vi "MGI Bezier Optimizer.vi"(0 "Sample Points":dbl[][](array[numeric]) format="%.2f", 1 "Substitution Matrix":dbl[][](array[numeric]) format="%.2f", 2 "Constant Vector":dbl[](array[numeric]) format="%.2f", 3 "Accuracy Limit":dbl=1e-08 format="%.3e", 4 "Start Vector":dbl[](array[numeric]) format="%.2f") -> (5 "Bezier Points":dbl[][](array[numeric]) format="%.2f", 6 "Log":dbl[][](array[numeric]) format="%.2f")   [LabVIEW 2020]
doc: "Modification of Downhill Simplex nD to perform modelling calculation and provide an interactive display.\n\nAuthored by David A. Moore\nsupport@mooregoodideas.com\nwww.mooregoodideas.com\n\nCopyright (c) 2010, Moore Good Ideas, Inc.\n\nAll rights reserved.\n\nRedistribution and use in source and binary forms, with or without modification, are permitted provided that the following conditions are met:\n\n * Redistributions of source code must retain the above copyright notice, this list of conditions and the following disclaimer.\n * Redistributions in binary form must reproduce the above copyright notice, this list of conditions and the following disclaimer in the documentation and/or other materials provided with the distribution.\n * Neither the name of Moore Good Ideas, Inc. nor the names of its contributors may be used to endorse or promote products derived from this software without specific prior written permission.\n\nTHIS SOFTWARE IS PROVIDED BY THE COPYRIGHT HOLDERS AND CONTRIBUTORS \"AS IS\" AND ANY EXPRESS OR IMPLIED WARRANTIES, INCLUDING, BUT NOT LIMITED TO, THE IMPLIED WARRANTIES OF MERCHANTABILITY AND FITNESS FOR A PARTICULAR PURPOSE ARE DISCLAIMED. IN NO EVENT SHALL THE COPYRIGHT OWNER OR CONTRIBUTORS BE LIABLE FOR ANY DIRECT, INDIRECT, INCIDENTAL, SPECIAL, EXEMPLARY, OR CONSEQUENTIAL DAMAGES (INCLUDING, BUT NOT LIMITED TO, PROCUREMENT OF SUBSTITUTE GOODS OR SERVICES; LOSS OF USE, DATA, OR PROFITS; OR BUSINESS INTERRUPTION) HOWEVER CAUSED AND ON ANY THEORY OF LIABILITY, WHETHER IN CONTRACT, STRICT LIABILITY, OR TORT (INCLUDING NEGLIGENCE OR OTHERWISE) ARISING IN ANY WAY OUT OF THE USE OF THIS SOFTWARE, EVEN IF ADVISED OF THE POSSIBILITY OF SUCH DAMAGE."
uses:
  <userlib>/_MGI/Bezier/MGI Bezier Fit Operation Enumeration.ctl
panel:
  in  "stop":bool
  out "XY Graph":T1(graph)
  in  "Iterations/plot":i32=1 min=1 max=100
  out "Accuracy":dbl=1e-08 format="%.3e"
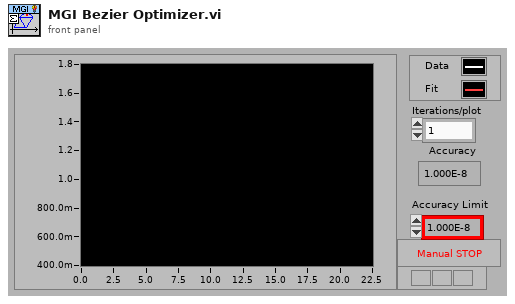
[diagram p1: front panel]
types:
  T1 = cluster{"Sample Points":dbl[], "Sample Points":dbl[]}[]
  T2 = typedef "MGI Bezier Fit Operation Enumeration.ctl" = enum16{"Initialize", "Test", "Read Curve", "Calc Bezier Points"}
  T3 = cluster{"Sample Points":dbl[], "Sample Points":dbl[]}
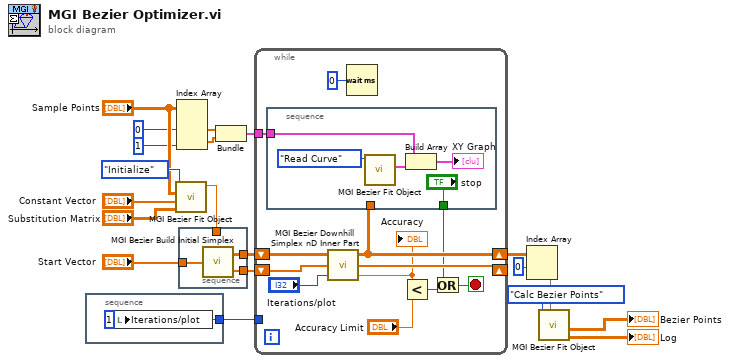
[diagram p0: block diagram]
diagram:
  n1 = stacked-sequence {
    tunnel: [w21] -> w16
    frame #0 {
      w21 = 1 ("Iterations/plot")
      n2 = local write "Iterations/plot"(w21) -> ()
    }
  }
  n3 = call <userlib>:"MGI Bezier Fit Object.vi"("Substitution Matrix[][]"="Substitution Matrix", "Constant Vector[]"="Constant Vector", "Sample Points[][]"="Sample Points", "Operation"=MGI_Bezier_Fit_Operation_Enumeration."Initialize") -> ("Error"=w1:dbl)  [unwired: 4 in, 3 out]
  n4 = Index Array(array="Sample Points", index (col) #1=0 ("Disabled Index (col)"), index (col) #2=1 ("Index (col)")) -> (element #1=w8:dbl[], element #2=w9:dbl[])  [unwired: 2 in]
  n5 = stacked-sequence {
    tunnel: [w24] -> w20
    tunnel: [w23] -> w19
    tunnel: "Start Vector" -> [w22]
    tunnel: w1 -> [_]
    frame #0 {
      n6 = call <userlib>:"MGI Bezier Build Initial Simplex.vi"("Start[]"=w22) -> ("Minimum before[][]"=w24:dbl[][], "f(Minimum) before[]"=w23:dbl[])
    }
  }
  n7 = Bundle("Sample Points"=w8, "Sample Points"=w9) -> (w7:T3)  [unwired: 1 in]
  n8 = while {
    tunnel: w7 -> [w25]
    tunnel: w16 -> [_]
    shift-left: w19 -> [w34]
    shift-right: [w33] -> _
    shift-left: w20 -> [w35]
    shift-right: [w32] -> w17
    stop <- w27 stop-if-true
    n9 = call <userlib>:"MGI Bezier Downhill Simplex nD Inner Part.vi"("Iterations"="Iterations/plot", "f(Minimum) Before[]"=w34, "Minimum Before[][]"=w35) -> ("Accuracy"=w31:dbl, "f(Minimum) After[]"=w33:dbl[], "Minimum After[][]"=w32:dbl[][])
    "Accuracy" <- w31
    n10 = stacked-sequence {
      tunnel: w32 -> [_]
      tunnel: ["stop"] -> w28
      tunnel: w25 -> [w38]
      frame #0 {
        n11 = call <userlib>:"MGI Bezier Fit Object.vi"("Operation"=MGI_Bezier_Fit_Operation_Enumeration."Read Curve") -> ("Model Curve"=w39:cluster{dbl[], dbl[]})  [unwired: 7 in, 3 out]
        n12 = Build Array(w38, w39) -> (→"XY Graph":T1)
      }
    }
    n13 = Wait (ms)(milliseconds to wait=u32 0) -> ()  [unwired: 1 out]
    n14 = Less?(x=w31, y="Accuracy Limit") -> (x < y?=w29:bool)
    n15 = Or(x=w28, y=w29) -> (x .or. y?=w27:bool)
  }
  n16 = Index Array(array=w17, index (row)=0) -> (element=w6:dbl[])  [unwired: 1 in]
  n17 = call <userlib>:"MGI Bezier Fit Object.vi"("Test Vector[]"=w6, "Operation"=MGI_Bezier_Fit_Operation_Enumeration."Calc Bezier Points") -> ("Log[][]"=→"Log":dbl[][], "Bezier Points[][]"=→"Bezier Points":dbl[][])  [unwired: 6 in, 2 out]
